vi "TDT-Wait For Device.vi"(0 "Output":T1, 9 "Timeout (ms)":dbl=5000.0, 11 "error in (no error)":errorcluster) -> (4 "Output thru":T1, 15 "error out":errorcluster)   [LabVIEW 2020]
uses:
  Typedefs/TDT-Output source.ctl
  Typedefs/TDT-Device ID.ctl
panel:
  out "GetStatus":i32
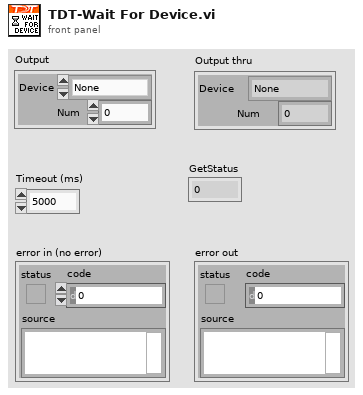
[diagram p1: front panel]
types:
  T1 = typedef "TDT-Output source.ctl" = cluster{"Device":T2, "Num":i32}
  T2 = typedef "TDT-Device ID.ctl" = enum16{"None", "PA5", "RP2", "RL2", "RA16", "RV8", "RX5", "RX6", "RX7", "RX8", "RZ2", "RZ5", "RZ6"}
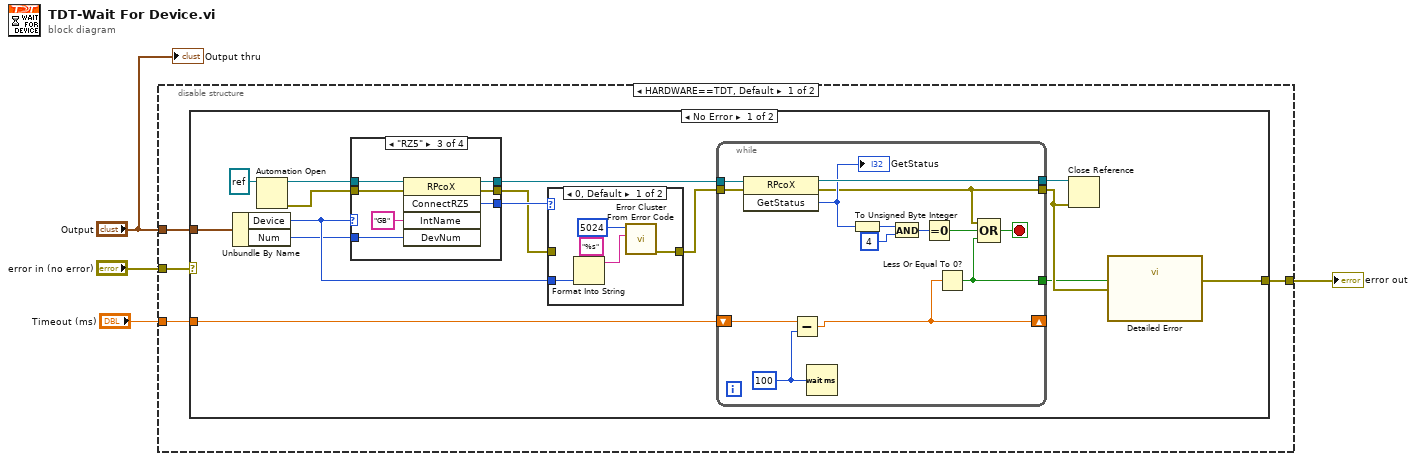
[diagram p0: block diagram]
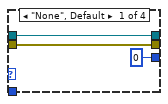
[diagram p2: hidden frame]
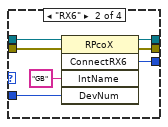
[diagram p3: hidden frame]
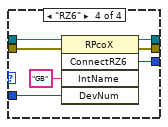
[diagram p4: hidden frame]
diagram:
  n1 = disable-structure shown="HARDWARE==TDT, Default" {
    disable-tunnel: "error in (no error)" -> [w6 w69]
    disable-tunnel: [w8 w69] -> w3
    disable-tunnel: "Output" -> [w7 _]
    disable-tunnel: "Timeout (ms)" -> [w5 _]
    frame condition #0 (active) {
      n2 = case shown="No Error" w6 {
        selector: w6 -> [_ w68]
        tunnel: [w9 w68] -> w8
        tunnel: w7 -> [w18 _]
        tunnel: w5 -> [w12 _]
        frame No Error {
          n3 = Unbundle By Name(w18) -> ("Device"=w17:T2, "Num"=w16:i32)
          n4 = Automation Open(Automation Refnum=refnum<k7> refnum ("RPCOXLib.RPcoX")) -> (Automation Refnum=w22:refnum<k7>, error out=w21:errorcluster)  [unwired: 3 in]
          n5 = case shown="\"RZ5\"" w17 {
            tunnel: w22 -> [w39 w47 w54 w61]
            tunnel: w21 -> [w40 w45 w52 w59]
            tunnel: [0 ("ConnectRX6") w44 w51 w58] -> w20
            tunnel: [w40 w43 w50 w57] -> w19
            tunnel: [w39 w42 w49 w56] -> w14
            tunnel: w16 -> [_ w41 w48 w55]
            frame "None", Default {
            }
            frame "RX6" {
              n6 = invoke class="RPcoX" method="ConnectRX6"(reference=w47, error in=w45, "IntName"="GB", "DevNum"=w41) -> (reference out=w42:refnum<k7>, error out=w43:errorcluster, "ConnectRX6"=w44:i32)  [unwired: 1 in, 2 out]
            }
            frame "RZ5" {
              n7 = invoke class="RPcoX" method="ConnectRZ5"(reference=w54, error in=w52, "IntName"="GB", "DevNum"=w48) -> (reference out=w49:refnum<k7>, error out=w50:errorcluster, "ConnectRZ5"=w51:i32)  [unwired: 1 in, 2 out]
            }
            frame "RZ6" {
              n8 = invoke class="RPcoX" method="ConnectRZ6"(reference=w61, error in=w59, "IntName"="GB", "DevNum"=w55) -> (reference out=w56:refnum<k7>, error out=w57:errorcluster, "ConnectRZ6"=w58:i32)  [unwired: 1 in, 2 out]
            }
          }
          n9 = case shown="0, Default" w20 {
            tunnel: w19 -> [_ w67]
            tunnel: [w65 w67] -> w13
            tunnel: w17 -> [w64 _]
            frame 0, Default {
              n10 = Format Into String(format string="%s", w64) -> (resulting string=w63:string)  [unwired: 2 in, 1 out]
              n11 = call <vilib>:"Error Cluster From Error Code.vi"("error message (\"\")"=w63, "error code (0)"=5024) -> ("error out"=w65:errorcluster)  [unwired: 7 in]
            }
            frame 1 {
            }
          }
          n12 = while {
            tunnel: w14 -> [w37]
            tunnel: w13 -> [w36]
            tunnel: [w35] -> w15
            shift-right: [w26] -> _
            shift-left: w12 -> [w29]
            tunnel: [w25] -> w10
            tunnel: [w24] -> w11
            stop <- w27 stop-if-true
            w28 = u32 100 ("milliseconds to wait")
            n13 = invoke class="RPcoX" method="GetStatus"(reference=w37, error in=w36) -> (reference out=w35:refnum<k7>, error out=w24:errorcluster, "GetStatus"=w34:i32)  [unwired: 1 in]
            "GetStatus" <- w34
            n14 = Subtract(x=w29, y=w28) -> (x-y=w26:dbl)
            n15 = Wait (ms)(milliseconds to wait=w28) -> ()  [unwired: 1 out]
            n16 = To Unsigned Byte Integer(number=w34) -> (unsigned 8bit integer=w33:u8)
            n17 = And(x=w33, y=u8 4) -> (x .and. y?=w31:u8)
            n18 = Equal To 0?(x=w31) -> (x = 0?=w30:bool)
            n19 = Less Or Equal To 0?(x=w26) -> (x <= 0?=w25:bool)
            n20 = Compound Arithmetic op=OR(w24, w30, w25) -> (w27:bool)
          }
          n21 = Close Reference(reference=w15, error in (no error)=w11) -> ()  [unwired: 1 out]
          n22 = call "Detailed Error"("Error?"=w10, "Primary"=w11) -> ("detailed error"=w9:errorcluster)  [unwired: 13 in]
        }
        frame Error {
        }
      }
    }
    frame condition #1 {
    }
  }
  "error out" <- w3
  "Output thru" <- "Output"
